vi "Test_allsw_PXI_Linux.vi"() -> (0 "pass":bool)   [LabVIEW 2019]
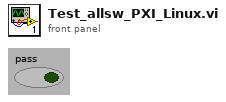
[diagram p1: front panel]
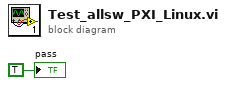
[diagram p0: block diagram]
diagram:
  "pass" <- TRUE
